vi "导出预设波形.vi"(10 "预设波形":dbl[][](array[numeric]), 11 "导出tdms文件参数":T1) -> ()   [LabVIEW 2018]
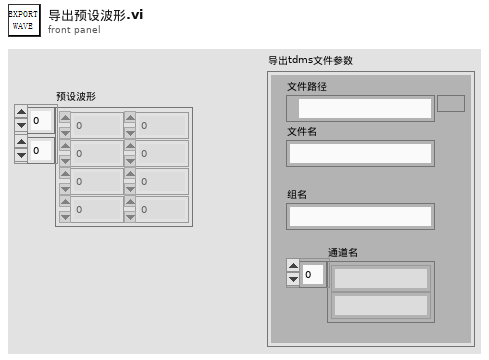
[diagram p1: front panel]
types:
  T1 = cluster{"组名":string, "通道名":string[], "文件路径":path, "文件名":string}
  T2 = enum16{"open", "open or create", "create or replace", "create", "open (read-only)"}
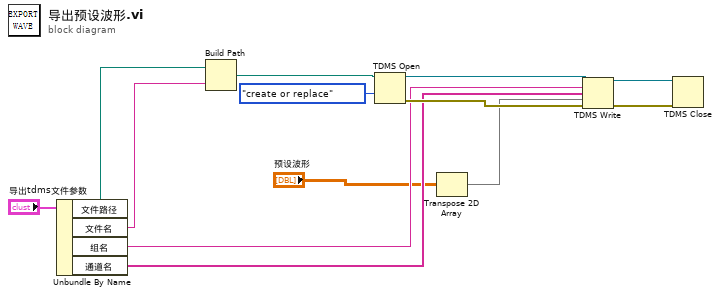
[diagram p0: block diagram]
diagram:
  n1 = Unbundle By Name("导出tdms文件参数") -> ("文件路径"=w6:path, "文件名"=w5:string, "组名"=w4:string, "通道名"=w3:string[])
  n2 = Build Path(base path=w6, name or relative path=w5) -> (appended path=w8:path)
  n3 = TDMS Open(10:T2."create or replace" ("operation (0:open)"), 11:w8) -> (0:w11:errorcluster, 3:w12:refnum<k34>)  [unwired: 5 in]
  n4 = Transpose 2D Array(2D array="预设波形") -> (transposed array=w1:dbl[][])
  n5 = TDMS Write(0:w12, 5:w4, 7:w3, 9:w1, 11:w11) -> (4:w10:refnum<k34>, 15:w9:errorcluster)  [unwired: 1 in, 2 out]
  n6 = TDMS Close(8:w9, 11:w10) -> ()  [unwired: 2 out]
